vi "Autonomous Independent.vi"() -> ()   [LabVIEW 2014]
doc: "This VI is called when autonomous begins, and will automatically be terminated when autonomous ends. You can carry out timed or sensor driven robot movement independently without needing to return to the caller."
uses:
  <vilib>/Rock Robotics/Network Tables/SD Read Number.vi
panel:
  in  "Desired Right Inches":dbl
  in  "Desired Left Inches":dbl
  # "Be sure to right-click and choose Data Operations>>Make Current Value default if you want to save the array values with the VI"
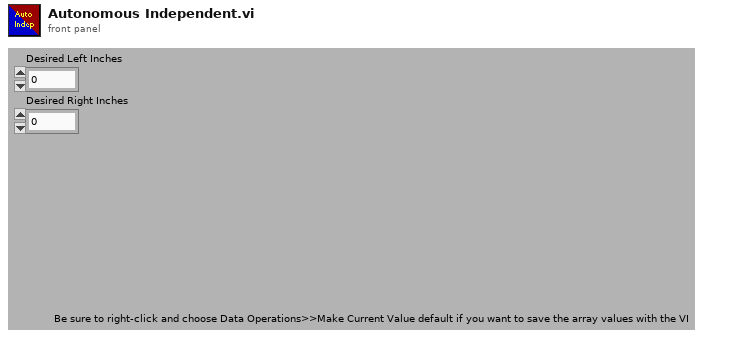
[diagram p1: front panel]
types:
  T1 = typedef "WPI_EncoderDevRef.ctl" = cluster{"DevStatus":errorcluster, "EncoderIndex":T2, "CounterIndex":T3, "DistancePerCount":dbl, "Decoding Type":T4}
  T2 = typedef "FPGA_EncoderIdx.ctl" = enum8{"Enc 0", "Enc 1", "Enc 2", "Enc 3", "Enc 4", "Enc 5", "Enc 6", "Enc 7", "Invalid"}
  T3 = typedef "FPGA_CounterCtrSystemIndex.ctl" = enum8{"Ctr 0", "Ctr 1", "Ctr 2", "Ctr 3", "Ctr 4", "Ctr 5", "Ctr 6", "Ctr 7", "Invalid"}
  T4 = typedef "WPI_EncoderType.ctl" = enum16{"1x", "2x", "4x"}
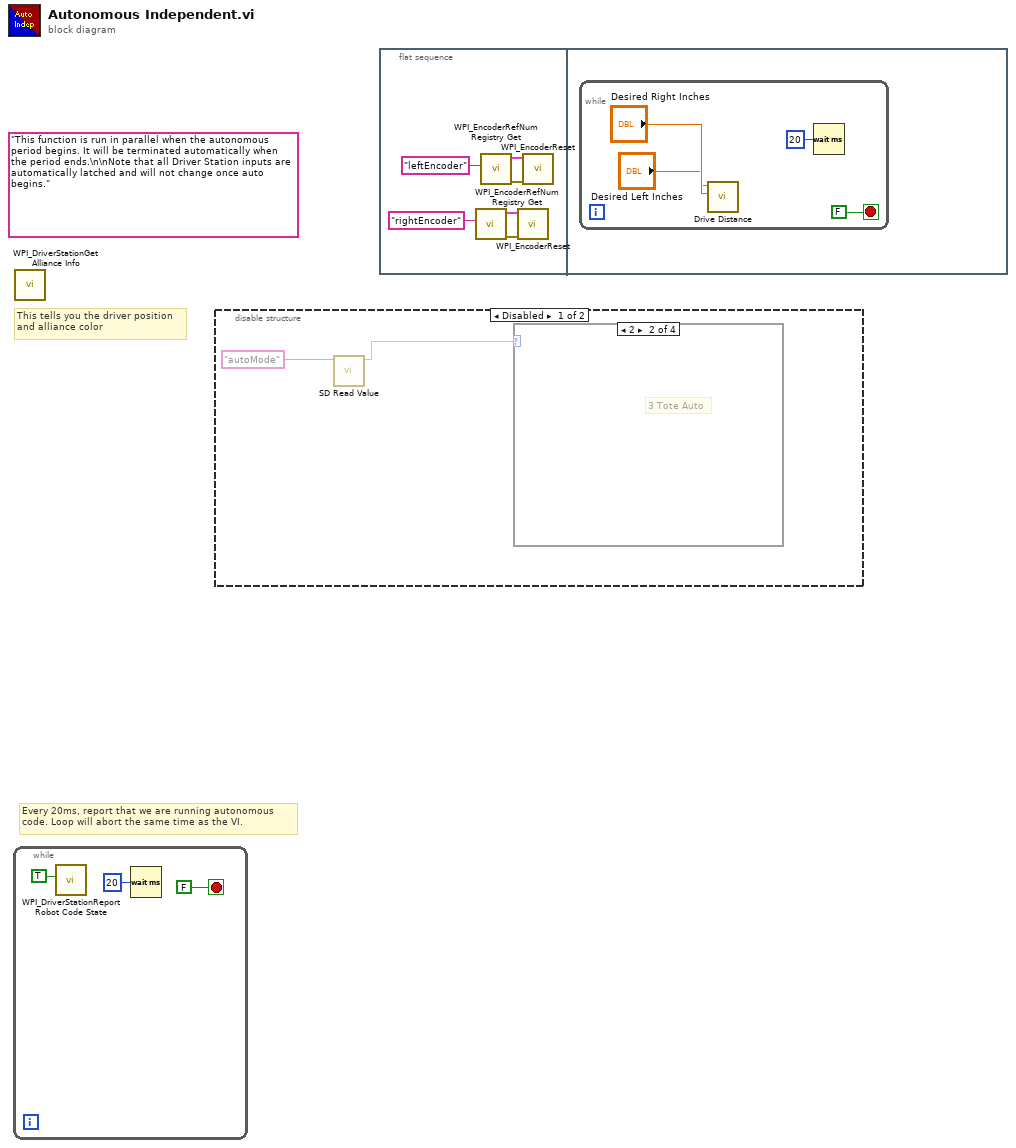
[diagram p0: block diagram]
diagram:
  (unwired) "This function is run in parallel when the autonomous period begins. It will be terminated automatically when the period ends.\n\nNote that all Driver Station inputs are automatically latched and will not change once auto begins."
  # "Every 20ms, report that we are running autonomous\ncode. Loop will abort the same time as the VI."
  # "This tells you the driver position\nand alliance color"
  n1 = while {
    stop <- FALSE stop-if-true
    n2 = call <vilib>:"WPI_DriverStationReport Robot Code State.vi"("Autonomous"=TRUE) -> ()  [unwired: 10 in, 1 out]
    n3 = Wait (ms)(milliseconds to wait=u32 20) -> ()  [unwired: 1 out]
  }
  n4 = call <vilib>:"WPI_DriverStationGet Alliance Info.vi"() -> ()  [unwired: 12 out]
  n5 = disable-structure shown="Disabled" {
    frame Disabled {
      n6 = call-poly <vilib>:"SD Read Value.vi"("Name"="autoMode") -> ("Numeric"=w4:dbl)  [unwired: 8 in, 2 out]
      n7 = case shown="2" w4 {
        frame 1 {
          # "1 Tote Auto"
        }
        frame 2 {
          # "3 Tote Auto"
        }
        frame 0 {
          # "Drive Forward Auto"
        }
        frame 3, Default {
        }
      }
    }
    frame Enabled {
    }
  }
  n8 = flat-sequence {
    frame #0 {
      n9 = call <vilib>:"WPI_EncoderRefNum Registry Get.vi"("refnum name"="rightEncoder") -> ("error out"=w6:errorcluster, "EncoderDevRef"=w7:T1)  [unwired: 9 in]
      n10 = call <vilib>:"WPI_EncoderRefNum Registry Get.vi"("refnum name"="leftEncoder") -> ("error out"=w11:errorcluster, "EncoderDevRef"=w10:T1)  [unwired: 9 in]
      n11 = call <vilib>:"WPI_EncoderReset.vi"("error in (no error)"=w6, "EncoderDevRef"=w7) -> ()  [unwired: 8 in, 2 out]
      n12 = call <vilib>:"WPI_EncoderReset.vi"("error in (no error)"=w11, "EncoderDevRef"=w10) -> ()  [unwired: 8 in, 2 out]
    }
    frame #1 {
      n13 = while {
        stop <- FALSE stop-if-true
        n14 = call "Drive Distance.vi"("Desired Right Inches"="Desired Right Inches", "Desired Left Inches"="Desired Left Inches") -> ()  [unwired: 10 in]
        n15 = Wait (ms)(milliseconds to wait=u32 20) -> ()  [unwired: 1 out]
      }
    }
  }
